vi "Query with 1D 64bit Integer Result.vi"(8 "error in (no error)":errorcluster, 10 "Query string":string, 11 "mysql in":refnum<class "mysql.lvclass">) -> (0 "error out":errorcluster, 2 "Result":i64[](array[numeric]), 3 "mysql out":refnum<class "mysql.lvclass">)   [LabVIEW 2020, in "mysql.lvlib" / "mysql.lvclass"]
uses:
  mysql.lvclass
  c7523bdb-939f-4a37-b533-c503b9257cc8.vi
  c7523bdb-939f-4a37-b533-c503b9257cc8.vi/81556f10-b1b4-4aff-b539-223732523efa.vi
  c7523bdb-939f-4a37-b533-c503b9257cc8.vi/abd803e7-4560-4929-a047-ec5595bacf32.vi
  private/Mysql command.vi
  private/Mysql data reader 1D I64.vi
  private/ping connection and reopen if needed.vi
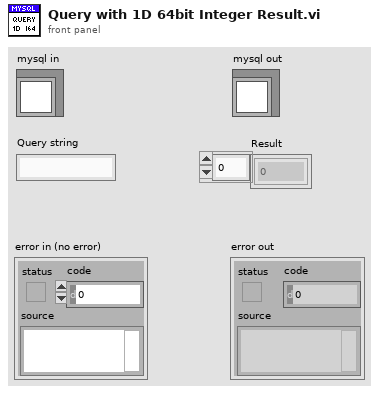
[diagram p1: front panel]
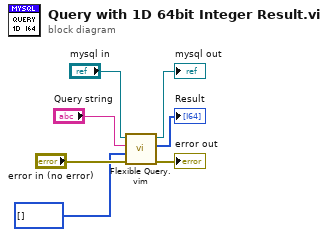
[diagram p0: block diagram]
diagram:
  n1 = call "Flexible Query.vim"("error in (no error)"="error in (no error)", "Type in"=i64[] [] ("Result 2"), "Query string"="Query string", "mysql in"="mysql in") -> ("error out"=→"error out":errorcluster, "Result"=→"Result":i64[], "mysql out"=→"mysql out":refnum<class "mysql.lvclass">)  [unwired: 5 in]
